vi "StartTrigger.vi"(8 "error in (no error)":errorcluster, 10 "trigger":string, 11 "PredictiveMaintenance in":refnum<class "PredictiveMaintenance.lvclass">) -> (0 "error out":errorcluster, 3 "PredictiveMaintenance out":refnum<class "PredictiveMaintenance.lvclass">)   [LabVIEW 2019, in "PredictiveMaintenance.lvlib" / "PredictiveMaintenance.lvclass"]
uses:
  PredictiveMaintenance.lvclass
  PredictiveMaintenance.lvclass/PredictiveMaintenance.ctl
  typedefs/Trigger_Data.ctl
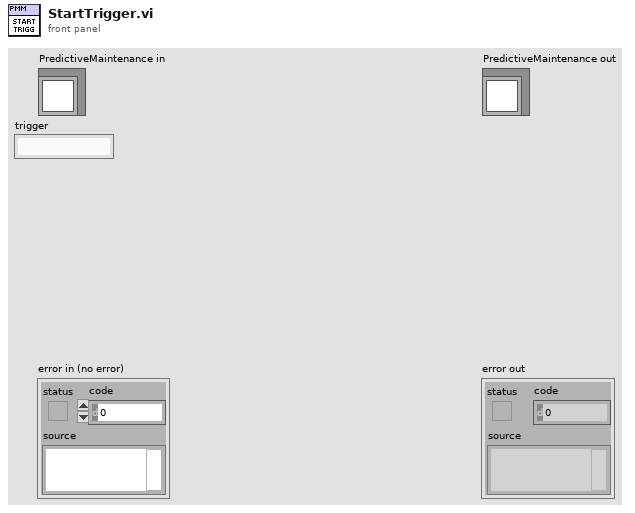
[diagram p1: front panel]
types:
  T1 = typedef "PredictiveMaintenance.lvlib/PredictiveMaintenance.lvclass/Trigger_Data.ctl" = cluster{"trigger":string, "curr_val (h)":dbl, "warn_limit (h)":dbl, "err_limit (h)":dbl, "running_timestamp":timestamp, "counter (h)":dbl}
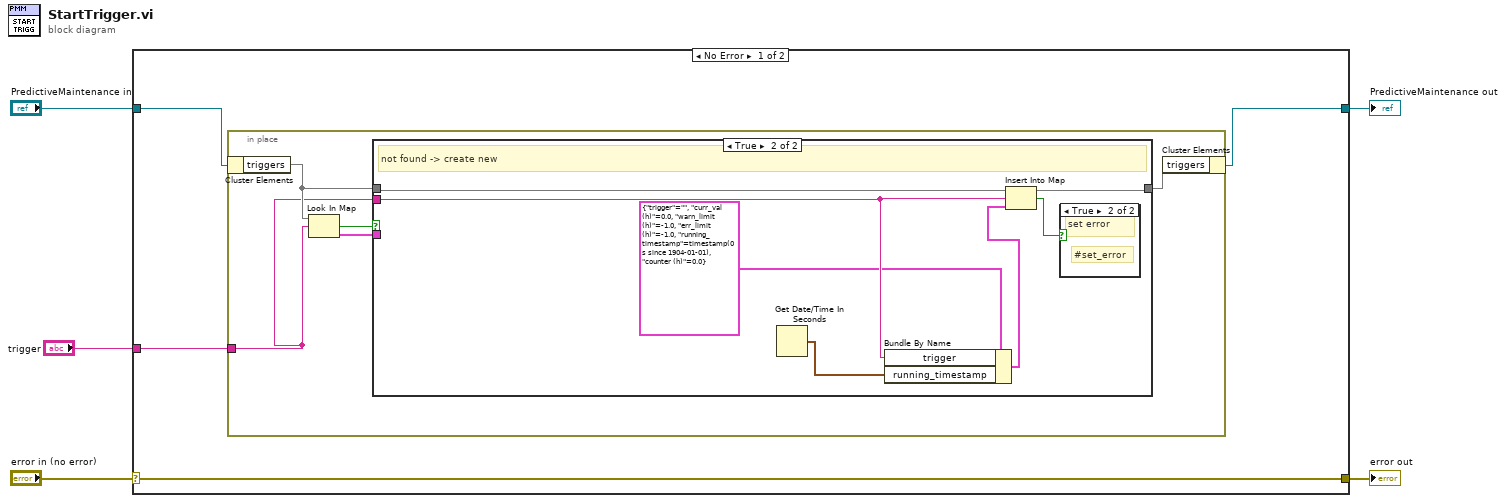
[diagram p0: block diagram]
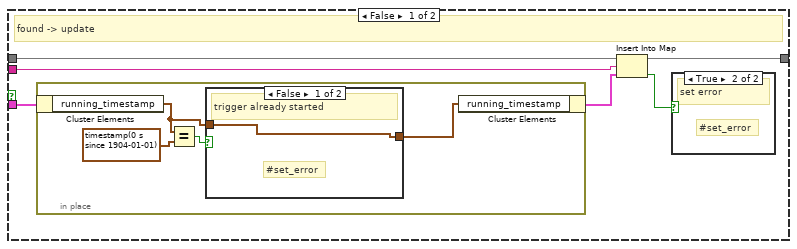
[diagram p2: hidden frame]
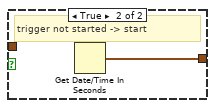
[diagram p4: hidden frame]
diagram:
  n1 = case shown="No Error" "error in (no error)" {
    selector: "error in (no error)" -> [w9 w35]
    tunnel: [w9 w35] -> w4
    tunnel: [w7 w34] -> w2
    tunnel: "PredictiveMaintenance in" -> [w8 w34]
    tunnel: "trigger" -> [w6 _]
    frame No Error {
      n2 = in-place {
        in-place-border: w6 -> [w10]
        n3 = in-place-cluster #1(w8) -> ("triggers"=w13:map{string, T1})
        n4 = Look In Map(map=w13, key=w10) -> (key not found?=w14:bool, value=w12:T1)  [unwired: 1 in]
        n5 = case shown="True" w14 {
          tunnel: w13 -> [w20 w33]
          tunnel: w12 -> [w16 _]
          tunnel: [w19 w32] -> w11
          tunnel: w10 -> [w18 w31]
          frame False {
            # "found -> update"
            n6 = in-place {
              n7 = in-place-cluster #2(w16) -> ("running_timestamp"=w21:timestamp)
              n8 = Equal?(x=w21, y=timestamp(0 s since 1904-01-01) ("current time")) -> (x = y?=w23:bool)
              n9 = case shown="False" w23 {
                tunnel: [w25 w26] -> w22
                tunnel: w21 -> [w25 _]
                frame False {
                  # "#set_error"
                  # "trigger already started"
                }
                frame True {
                  # "trigger not started -> start"
                  n10 = Get Date/Time In Seconds() -> (seconds since 1Jan1904=w26:timestamp)
                }
              }
              n11 = in-place-cluster #2("running_timestamp"=w22) -> (w15:T1)
            }
            n12 = Insert Into Map(map in=w20, key=w18, value=w15) -> (map out=w19:map{string, T1}, value unchanged?=w17:bool)  [unwired: 1 out]
            n13 = case shown="True" w17 {
              frame False {
              }
              frame True {
                # "#set_error"
                # "set error"
              }
            }
          }
          frame True {
            # "not found -> create new"
            n14 = Get Date/Time In Seconds() -> (seconds since 1Jan1904=w28:timestamp)
            n15 = Bundle By Name(cluster=T1 {"trigger"="", "curr_val (h)"=0.0, "warn_limit (h)"=-1.0, "err_limit (h)"=-1.0, "running_timestamp"=timestamp(0 s since 1904-01-01), "counter (h)"=0.0} ("event_data"), "trigger"=w31, "running_timestamp"=w28) -> (w27:T1)
            n16 = Insert Into Map(map in=w33, key=w31, value=w27) -> (map out=w32:map{string, T1}, key already included?=w30:bool)  [unwired: 1 out]
            n17 = case shown="True" w30 {
              frame False {
              }
              frame True {
                # "#set_error"
                # "set error"
              }
            }
          }
        }
        n18 = in-place-cluster #1("triggers"=w11) -> (w7:refnum<class "PredictiveMaintenance.lvclass">)
      }
    }
    frame Error {
    }
  }
  "error out" <- w4
  "PredictiveMaintenance out" <- w2
